vi "WCA_GET_PLL.vi"(0 "Cartridge Band":u32=10, 1 "Slave Node in":cluster{"Address":i16, "Serial Number":i8[]}={"Address"=19, "Serial Number"=[16, 71, 55, 76, 1, 8, 0, -15]} {"Serial Number" format="%.0x"; "Address" format="%.0x"}, 2 "ObjHandle in":u32, 11 "error in (no error)":errorcluster) -> (4 "ObjHandle out":u32=92930112, 8 "GET_PLL":T1={"PLL_ASSY_T"=35.217285, "PLL_REF_TOT_P"=-2.1250916, "PLL_IF_TOT_P"=-4.8457336, "PLL_CORR_V"=-0.14390425, "PLL_LOCK_V"=5.097532, "PLL_5V_SUPPLY_V"=18.560791, "Temp_TF"=TRUE, "PLL Ref Pwr_TF"=TRUE, "IF Pwr_TF"=TRUE, "PLL Corr_TF"=TRUE, "PLL Lock V_TF"=TRUE, "PLL Nominal_TF"=TRUE}, 15 "error out":errorcluster)   [LabVIEW 2017]
uses:
  WCA_Global.vi
panel:
  # "Node Address"
  # "Serial Number"
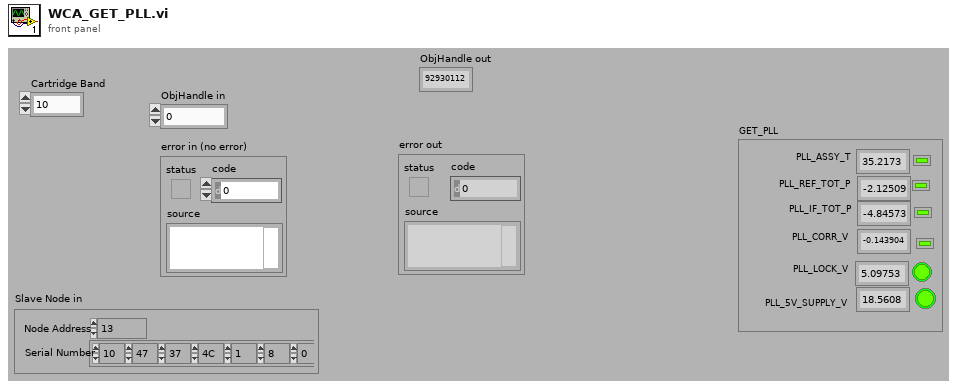
[diagram p1: front panel]
types:
  T1 = cluster{"PLL_ASSY_T":sgl, "PLL_REF_TOT_P":sgl, "PLL_IF_TOT_P":sgl, "PLL_CORR_V":sgl, "PLL_LOCK_V":sgl, "PLL_5V_SUPPLY_V":sgl, "Temp_TF":bool, "PLL Ref Pwr_TF":bool, "IF Pwr_TF":bool, "PLL Corr_TF":bool, "PLL Lock V_TF":bool, "PLL Nominal_TF":bool}
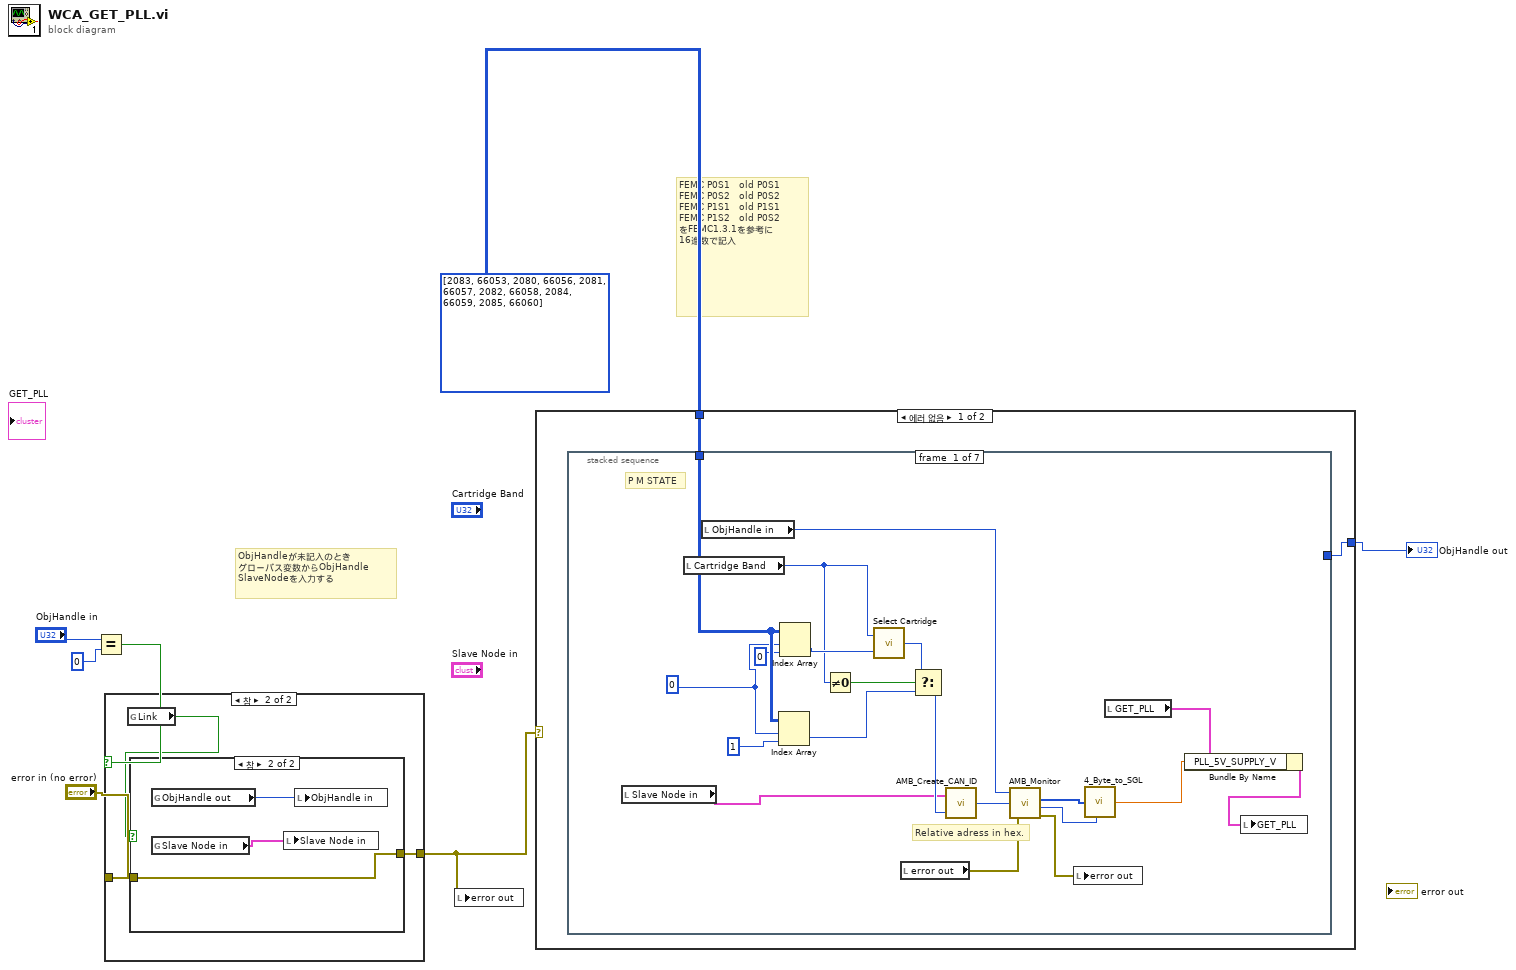
[diagram p0: block diagram]
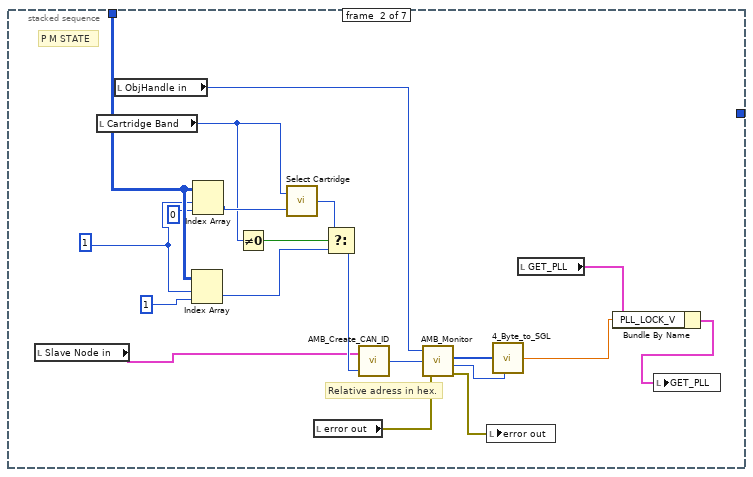
[diagram p2: hidden frame]
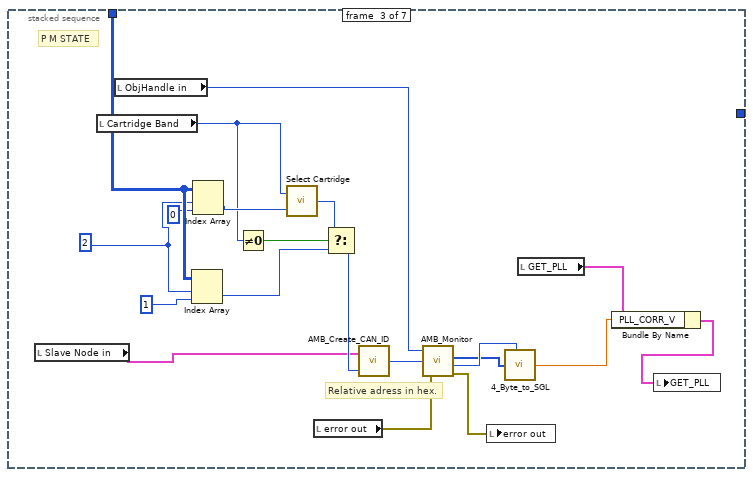
[diagram p3: hidden frame]
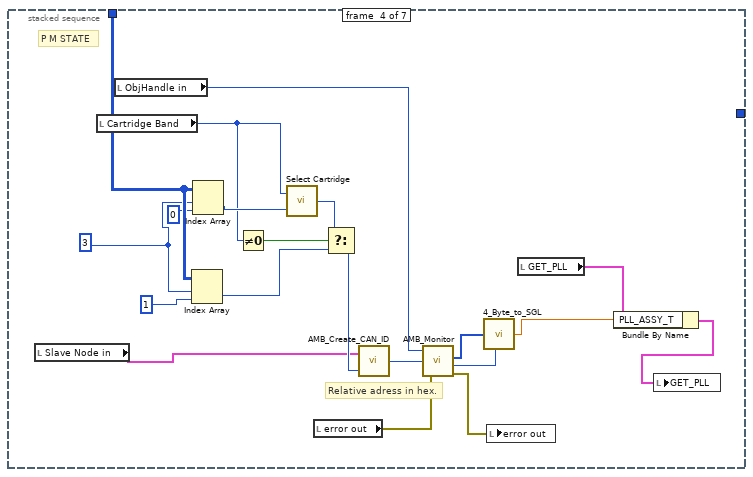
[diagram p4: hidden frame]
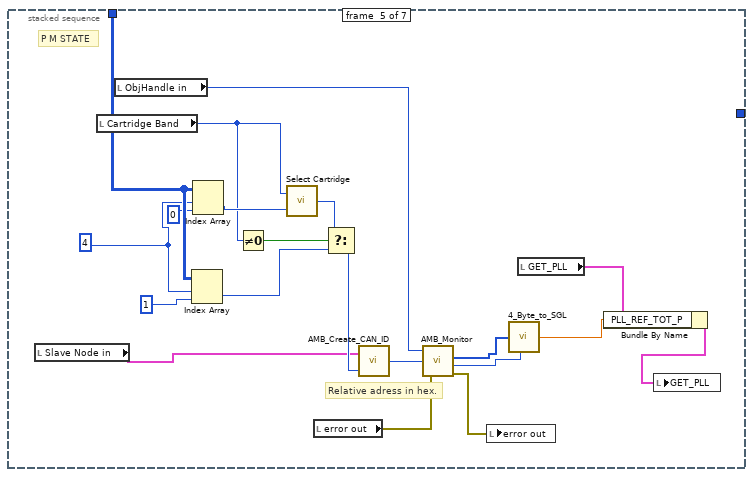
[diagram p5: hidden frame]
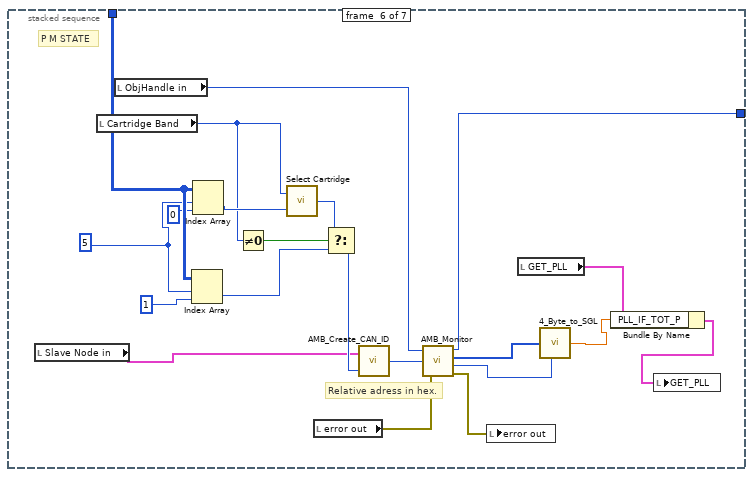
[diagram p6: hidden frame]
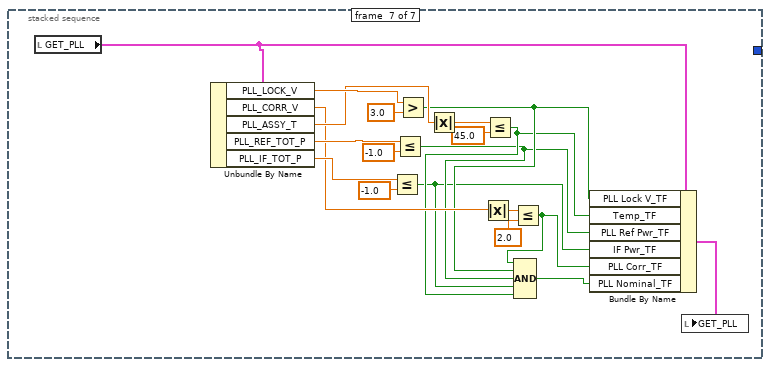
[diagram p7: hidden frame]
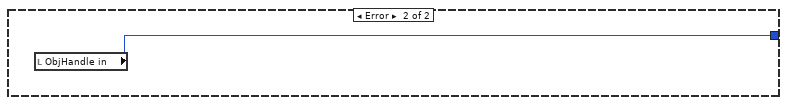
[diagram p8: hidden frame]
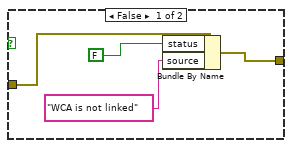
[diagram p10: hidden frame]
diagram:
  # "ObjHandleが未記入のとき\nグローバス変数からObjHandle\nSlaveNodeを入力する"
  # "FEMC P0S1   old P0S1\nFEMC P0S2   old P0S2\nFEMC P1S1   old P1S1\nFEMC P1S2   old P0S2\nをFEMC1.3.1を参考に\n16進数で記入"
  n1 = Equal?(x="ObjHandle in", y=0) -> (x = y?=w5:bool)
  n2 = case shown="참" w5 {
    tunnel: "error in (no error)" -> [w8 w11]
    tunnel: [w8 w10] -> w3
    frame False {
    }
    frame True {
      n3 = global read "WCA_Global.vi" "Link"() -> (w9:bool)
      n4 = case shown="참" w9 {
        tunnel: w11 -> [w15 w16]
        tunnel: [w12 w16] -> w10
        frame False {
          n5 = Bundle By Name(cluster=w15, "status"=FALSE, "source"="WCA is not linked") -> (w12:errorcluster)
        }
        frame True {
          n6 = global read "WCA_Global.vi" "ObjHandle out"() -> (w18:u32)
          n7 = global read "WCA_Global.vi" "Slave Node in"() -> (w17:cluster{"Address":i16, "Serial Number":i8[]})
          n8 = local write "Slave Node in"(w17) -> ()
          n9 = local write "ObjHandle in"(w18) -> ()
        }
      }
    }
  }
  n10 = local write "error out"(w3) -> ()
  n11 = case shown="에러 없음" w3 {
    tunnel: [w19 w162] -> w2
    tunnel: i32[][] [[2083, 66053], [2080, 66056], [2081, 66057], [2082, 66058], [2084, 66059], [2085, 66060]] -> [w20 _]
    frame No Error {
      n12 = stacked-sequence {
        tunnel: w20 -> [w40 w60 w80 w100 w120 w141 _]
        tunnel: [_ _ _ _ _ w124 _] -> w19
        frame #0 {
          w25 = 0
          # "Relative adress in hex."
          # "P M STATE"
          n13 = local read "Slave Node in"() -> (w24:cluster{"Address":i16, "Serial Number":i8[]})
          n14 = local read "Cartridge Band"() -> (w26:u32)
          n15 = local read "ObjHandle in"() -> (w36:u32)
          n16 = Index Array(array=w40, index (row)=w25, index (col)=1) -> (element=w35:i32)
          n17 = Index Array(array=w40, index (row)=w25, index (col)=0) -> (element=w34:i32)
          n18 = Not Equal To 0?(x=w26) -> (x != 0?=w37:bool)
          n19 = call "Select Cartridge.vi"("Relative Address in"=w34, "Cartridge band"=w26) -> ("Relative Address out"=w38:u32)
          n20 = local read "error out"() -> (w28:errorcluster)
          n21 = Select(t=w38, s=w37, f=w35) -> (s? t:f=w39:u32)
          n22 = call "AMB_Create_CAN_ID.vi"("Relative Address in"=w39, "Slave Node in"=w24) -> ("CAN ID out"=w31:u32)
          n23 = call "AMB_Monitor.vi"("ObjHandle in"=w36, "CAN ID in"=w31, "error in"=w28) -> ("Data Array out"=w23:u8[], "Data Length out"=w22:u8, "error out"=w27:errorcluster)  [unwired: 1 out]
          n24 = local write "error out"(w27) -> ()
          n25 = call "4_Byte_to_SGL.vi"("Array of 4 bytes"=w23, "number of valid bytes"=w22) -> ("Number"=w21:sgl)  [unwired: 1 out]
          n26 = local read "GET_PLL"() -> (w30:T1)
          n27 = Bundle By Name(cluster=w30, "PLL_5V_SUPPLY_V"=w21) -> (w29:T1)
          n28 = local write "GET_PLL"(w29) -> ()
        }
        frame #1 {
          w45 = 1
          # "Relative adress in hex."
          # "P M STATE"
          n29 = local read "Slave Node in"() -> (w44:cluster{"Address":i16, "Serial Number":i8[]})
          n30 = local read "Cartridge Band"() -> (w46:u32)
          n31 = local read "ObjHandle in"() -> (w56:u32)
          n32 = Index Array(array=w60, index (row)=w45, index (col)=1) -> (element=w55:i32)
          n33 = Index Array(array=w60, index (row)=w45, index (col)=0) -> (element=w54:i32)
          n34 = Not Equal To 0?(x=w46) -> (x != 0?=w57:bool)
          n35 = call "Select Cartridge.vi"("Relative Address in"=w54, "Cartridge band"=w46) -> ("Relative Address out"=w58:u32)
          n36 = local read "error out"() -> (w48:errorcluster)
          n37 = Select(t=w58, s=w57, f=w55) -> (s? t:f=w59:u32)
          n38 = call "AMB_Create_CAN_ID.vi"("Relative Address in"=w59, "Slave Node in"=w44) -> ("CAN ID out"=w51:u32)
          n39 = call "AMB_Monitor.vi"("ObjHandle in"=w56, "CAN ID in"=w51, "error in"=w48) -> ("Data Array out"=w43:u8[], "Data Length out"=w42:u8, "error out"=w47:errorcluster)  [unwired: 1 out]
          n40 = local write "error out"(w47) -> ()
          n41 = call "4_Byte_to_SGL.vi"("Array of 4 bytes"=w43, "number of valid bytes"=w42) -> ("Number"=w41:sgl)  [unwired: 1 out]
          n42 = local read "GET_PLL"() -> (w50:T1)
          n43 = Bundle By Name(cluster=w50, "PLL_LOCK_V"=w41) -> (w49:T1)
          n44 = local write "GET_PLL"(w49) -> ()
        }
        frame #2 {
          w65 = 2
          # "Relative adress in hex."
          # "P M STATE"
          n45 = local read "Slave Node in"() -> (w64:cluster{"Address":i16, "Serial Number":i8[]})
          n46 = local read "Cartridge Band"() -> (w66:u32)
          n47 = local read "ObjHandle in"() -> (w76:u32)
          n48 = Index Array(array=w80, index (row)=w65, index (col)=1) -> (element=w75:i32)
          n49 = Index Array(array=w80, index (row)=w65, index (col)=0) -> (element=w74:i32)
          n50 = Not Equal To 0?(x=w66) -> (x != 0?=w77:bool)
          n51 = call "Select Cartridge.vi"("Relative Address in"=w74, "Cartridge band"=w66) -> ("Relative Address out"=w78:u32)
          n52 = local read "error out"() -> (w68:errorcluster)
          n53 = Select(t=w78, s=w77, f=w75) -> (s? t:f=w79:u32)
          n54 = call "AMB_Create_CAN_ID.vi"("Relative Address in"=w79, "Slave Node in"=w64) -> ("CAN ID out"=w71:u32)
          n55 = call "AMB_Monitor.vi"("ObjHandle in"=w76, "CAN ID in"=w71, "error in"=w68) -> ("Data Array out"=w62:u8[], "Data Length out"=w63:u8, "error out"=w67:errorcluster)  [unwired: 1 out]
          n56 = local write "error out"(w67) -> ()
          n57 = call "4_Byte_to_SGL.vi"("Array of 4 bytes"=w62, "number of valid bytes"=w63) -> ("Number"=w61:sgl)  [unwired: 1 out]
          n58 = local read "GET_PLL"() -> (w70:T1)
          n59 = Bundle By Name(cluster=w70, "PLL_CORR_V"=w61) -> (w69:T1)
          n60 = local write "GET_PLL"(w69) -> ()
        }
        frame #3 {
          w85 = 3
          # "Relative adress in hex."
          # "P M STATE"
          n61 = local read "Slave Node in"() -> (w84:cluster{"Address":i16, "Serial Number":i8[]})
          n62 = local read "Cartridge Band"() -> (w86:u32)
          n63 = local read "ObjHandle in"() -> (w96:u32)
          n64 = Index Array(array=w100, index (row)=w85, index (col)=1) -> (element=w95:i32)
          n65 = Index Array(array=w100, index (row)=w85, index (col)=0) -> (element=w94:i32)
          n66 = Not Equal To 0?(x=w86) -> (x != 0?=w97:bool)
          n67 = call "Select Cartridge.vi"("Relative Address in"=w94, "Cartridge band"=w86) -> ("Relative Address out"=w98:u32)
          n68 = local read "error out"() -> (w88:errorcluster)
          n69 = Select(t=w98, s=w97, f=w95) -> (s? t:f=w99:u32)
          n70 = call "AMB_Create_CAN_ID.vi"("Relative Address in"=w99, "Slave Node in"=w84) -> ("CAN ID out"=w91:u32)
          n71 = call "AMB_Monitor.vi"("ObjHandle in"=w96, "CAN ID in"=w91, "error in"=w88) -> ("Data Array out"=w83:u8[], "Data Length out"=w82:u8, "error out"=w87:errorcluster)  [unwired: 1 out]
          n72 = call "4_Byte_to_SGL.vi"("Array of 4 bytes"=w83, "number of valid bytes"=w82) -> ("Number"=w81:sgl)  [unwired: 1 out]
          n73 = local write "error out"(w87) -> ()
          n74 = local read "GET_PLL"() -> (w90:T1)
          n75 = Bundle By Name(cluster=w90, "PLL_ASSY_T"=w81) -> (w89:T1)
          n76 = local write "GET_PLL"(w89) -> ()
        }
        frame #4 {
          w105 = 4
          # "Relative adress in hex."
          # "P M STATE"
          n77 = local read "Slave Node in"() -> (w104:cluster{"Address":i16, "Serial Number":i8[]})
          n78 = local read "Cartridge Band"() -> (w106:u32)
          n79 = local read "ObjHandle in"() -> (w116:u32)
          n80 = Index Array(array=w120, index (row)=w105, index (col)=1) -> (element=w115:i32)
          n81 = Index Array(array=w120, index (row)=w105, index (col)=0) -> (element=w114:i32)
          n82 = Not Equal To 0?(x=w106) -> (x != 0?=w117:bool)
          n83 = call "Select Cartridge.vi"("Relative Address in"=w114, "Cartridge band"=w106) -> ("Relative Address out"=w118:u32)
          n84 = local read "error out"() -> (w108:errorcluster)
          n85 = Select(t=w118, s=w117, f=w115) -> (s? t:f=w119:u32)
          n86 = call "AMB_Create_CAN_ID.vi"("Relative Address in"=w119, "Slave Node in"=w104) -> ("CAN ID out"=w111:u32)
          n87 = call "AMB_Monitor.vi"("ObjHandle in"=w116, "CAN ID in"=w111, "error in"=w108) -> ("Data Array out"=w103:u8[], "Data Length out"=w102:u8, "error out"=w107:errorcluster)  [unwired: 1 out]
          n88 = local write "error out"(w107) -> ()
          n89 = call "4_Byte_to_SGL.vi"("Array of 4 bytes"=w103, "number of valid bytes"=w102) -> ("Number"=w101:sgl)  [unwired: 1 out]
          n90 = local read "GET_PLL"() -> (w110:T1)
          n91 = Bundle By Name(cluster=w110, "PLL_REF_TOT_P"=w101) -> (w109:T1)
          n92 = local write "GET_PLL"(w109) -> ()
        }
        frame #5 {
          w126 = 5
          # "Relative adress in hex."
          # "P M STATE"
          n93 = local read "Slave Node in"() -> (w125:cluster{"Address":i16, "Serial Number":i8[]})
          n94 = local read "Cartridge Band"() -> (w127:u32)
          n95 = local read "ObjHandle in"() -> (w137:u32)
          n96 = Index Array(array=w141, index (row)=w126, index (col)=1) -> (element=w136:i32)
          n97 = Index Array(array=w141, index (row)=w126, index (col)=0) -> (element=w135:i32)
          n98 = Not Equal To 0?(x=w127) -> (x != 0?=w138:bool)
          n99 = call "Select Cartridge.vi"("Relative Address in"=w135, "Cartridge band"=w127) -> ("Relative Address out"=w139:u32)
          n100 = local read "error out"() -> (w129:errorcluster)
          n101 = Select(t=w139, s=w138, f=w136) -> (s? t:f=w140:u32)
          n102 = call "AMB_Create_CAN_ID.vi"("Relative Address in"=w140, "Slave Node in"=w125) -> ("CAN ID out"=w132:u32)
          n103 = call "AMB_Monitor.vi"("ObjHandle in"=w137, "CAN ID in"=w132, "error in"=w129) -> ("ObjHandle out"=w124:u32, "Data Array out"=w123:u8[], "Data Length out"=w122:u8, "error out"=w128:errorcluster)
          n104 = local write "error out"(w128) -> ()
          n105 = local read "GET_PLL"() -> (w131:T1)
          n106 = call "4_Byte_to_SGL.vi"("Array of 4 bytes"=w123, "number of valid bytes"=w122) -> ("Number"=w121:sgl)  [unwired: 1 out]
          n107 = Bundle By Name(cluster=w131, "PLL_IF_TOT_P"=w121) -> (w130:T1)
          n108 = local write "GET_PLL"(w130) -> ()
        }
        frame #6 {
          n109 = local read "GET_PLL"() -> (w149:T1)
          n110 = Unbundle By Name(w149) -> ("PLL_LOCK_V"=w154:sgl, "PLL_CORR_V"=w150:sgl, "PLL_ASSY_T"=w153:sgl, "PLL_REF_TOT_P"=w152:sgl, "PLL_IF_TOT_P"=w151:sgl)
          n111 = Less Or Equal?(x=w151, y=sgl -1.0) -> (x <= y?=w145:bool)
          n112 = Less Or Equal?(x=w152, y=sgl -1.0) -> (x <= y?=w146:bool)
          n113 = Greater?(x=w154, y=sgl 3.0) -> (0:w148:bool)
          n114 = Absolute Value(x=w153) -> (abs(x)=w156:sgl)
          n115 = Absolute Value(x=w150) -> (abs(x)=w158:sgl)
          n116 = Less Or Equal?(x=w156, y=sgl 45.0) -> (x <= y?=w147:bool)
          n117 = Less Or Equal?(x=w158, y=sgl 2.0) -> (x <= y?=w142:bool)
          n118 = Compound Arithmetic op=AND(w142, w148, w146, w145, w147) -> (w144:bool)
          n119 = Bundle By Name(cluster=w149, "PLL Lock V_TF"=w148, "Temp_TF"=w147, "PLL Ref Pwr_TF"=w146, "IF Pwr_TF"=w145, "PLL Corr_TF"=w142, "PLL Nominal_TF"=w144) -> (w143:T1)
          n120 = local write "GET_PLL"(w143) -> ()
        }
      }
    }
    frame Error {
      n121 = local read "ObjHandle in"() -> (w162:u32)
    }
  }
  "ObjHandle out" <- w2
